vi "GaGe4_QueryChannelParameters .vi"(8 "error in (no error)":errorcluster, 10 "Input settings":T1(array[cluster]), 11 "Handle Cluster in":T2) -> (0 "error out":errorcluster, 2 "Input settings out":T1(array[cluster]))   [LabVIEW 2015]
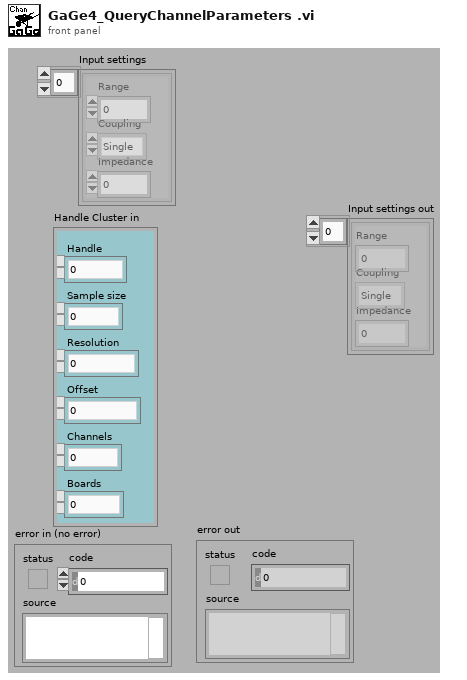
[diagram p1: front panel]
types:
  T1 = cluster{"Range":dbl, "Coupling":enum16{"Single", "Differen"}, "Impedance":dbl}[]
  T2 = cluster{"Handle":u32, "Sample size":u32, "Resolution":i32, "Offset":i32, "Channels":u32, "Boards":u32}
  T3 = cluster{"Range":dbl, "Coupling":enum16{"Single", "Differen"}, "Impedance":dbl}
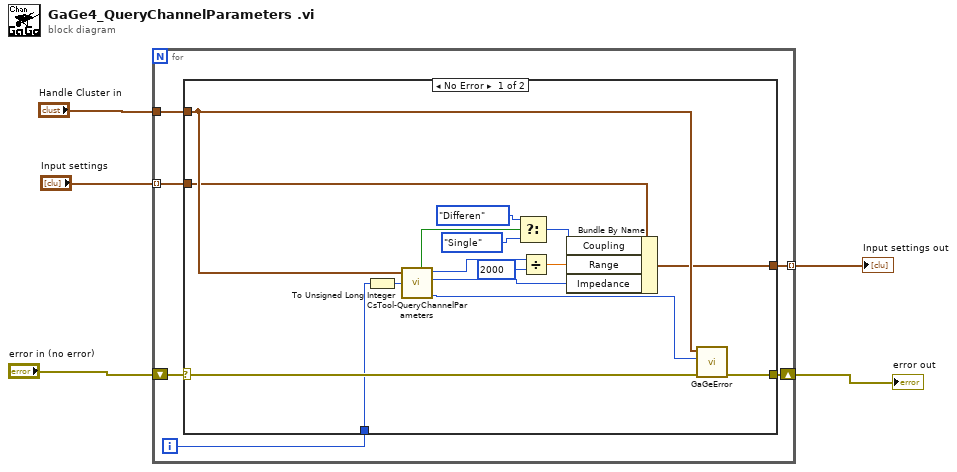
[diagram p0: block diagram]
diagram:
  n1 = for {
    tunnel: "Handle Cluster in" -> [w9]
    shift-right: [w10] -> w4
    shift-left: "error in (no error)" -> [w11]
    tunnel: "Input settings" -> [w7] mode=indexing
    tunnel: [w6] -> w1 mode=indexing
    i -> [w8]
    n2 = case shown="No Error" w11 {
      selector: w11 -> [w27 w29]
      tunnel: [w26 w29] -> w10
      tunnel: w9 -> [w24 _]
      tunnel: w8 -> [w22 _]
      tunnel: w7 -> [w21 w28]
      tunnel: [w17 w28] -> w6
      frame No Error {
        n3 = To Unsigned Long Integer(number=w22) -> (unsigned 32bit integer=w23:u32)
        n4 = call "CsTool-QueryChannelParameters.vi"("Channel"=w23, "Handle Cluster"=w24) -> ("Error Code"=w25:i32, "Impedance"=w16:u32, "Differential Input"=w18:bool, "Range (mV)"=w13:u32)  [unwired: 3 out]
        n5 = Select(t=enum16{"Single", "Differen"}."Differen" ("Coupling"), s=w18, f=enum16{"Single", "Differen"}."Single" ("Coupling")) -> (s? t:f=w15:enum16{"Single", "Differen"})
        n6 = Divide(x=w13, y=u32 2000) -> (x/y=w14:dbl)
        n7 = Bundle By Name(cluster=w21, "Coupling"=w15, "Range"=w14, "Impedance"=w16) -> (w17:T3)
        n8 = call "GaGeError.vi"("error in (no error)"=w27, "Error Code"=w25, "Handle Cluster"=w24) -> ("error out"=w26:errorcluster)  [unwired: 3 in, 5 out]
      }
      frame Error {
      }
    }
  }
  "error out" <- w4
  "Input settings out" <- w1
